vi "Read Socket.lvclass.vi"(8 "error in (no error)":errorcluster, 11 "Communication Manager in":refnum<class "Communication Manager.lvclass">) -> (0 "error out":errorcluster, 2 "Socket.lvclass":refnum<class "Socket.lvclass">, 3 "Communication Manager out":refnum<class "Communication Manager.lvclass">)   [LabVIEW 2018, in "Communication Manager.lvclass"]
uses:
  Communication Manager.lvclass
  Socket/Socket.lvclass
  Communication Manager.lvclass/Communication Manager.ctl
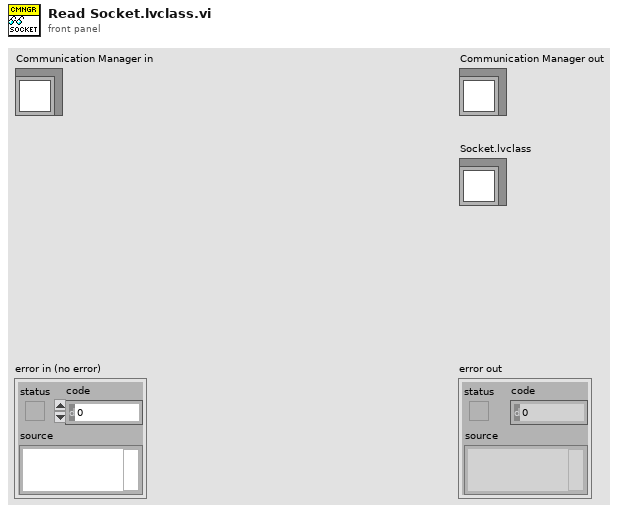
[diagram p1: front panel]
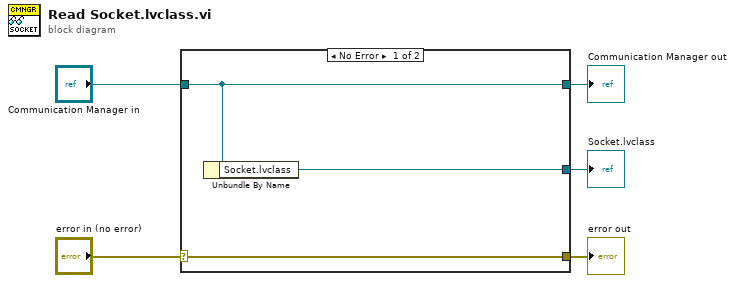
[diagram p0: block diagram]
diagram:
  n1 = case shown="No Error" "error in (no error)" {
    selector: "error in (no error)" -> [w8 w9]
    tunnel: [w8 w9] -> w4
    tunnel: [w7 w10] -> w2
    tunnel: "Communication Manager in" -> [w7 w10]
    tunnel: [w6 _] -> w1
    frame No Error {
      n2 = Unbundle By Name(w7) -> ("Socket.lvclass"=w6:refnum<class "Socket.lvclass">)
    }
    frame Error {
    }
  }
  "error out" <- w4
  "Communication Manager out" <- w2
  "Socket.lvclass" <- w1
